vi "Insert Reference.vi"(4 "Error In":errorcluster, 6 "Plugin Name":T1, 7 "WFChart Refnum":refnum<vi>) -> (0 "Error Out":errorcluster)   [LabVIEW 2015, in "Plugin Chart References.lvlib"]
uses:
  Plugin Chart References.lvlib
  _libraries/Startup Processes/_typedefs/Subpanel Names.ctl
  _libraries/Startup Processes/Startup Processes.lvlib
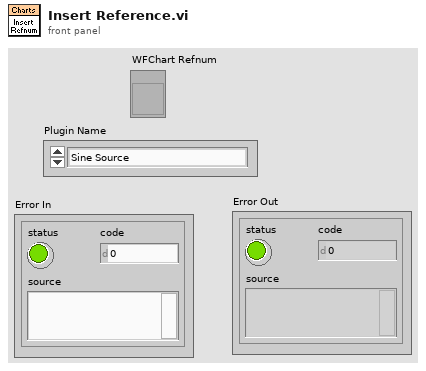
[diagram p1: front panel]
types:
  T1 = typedef "Startup Processes.lvlib/Subpanel Names.ctl" = enum16{"Sine Source", "Ramp Source", "Hen House TC", "Dog House TC", "Out House TC"}
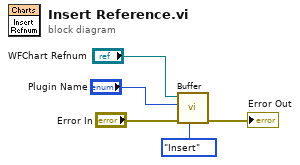
[diagram p0: block diagram]
diagram:
  n1 = call "Buffer.vi"("Function"=enum16{"Read", "Insert"}."Insert", "Error In"="Error In", "Plugin Name"="Plugin Name", "Reference In"="WFChart Refnum") -> ("Error Out"=→"Error Out":errorcluster)  [unwired: 3 in, 1 out]
